vi "Generate Function Call Argument Info.vi"(8 "error in (no error)":errorcluster, 11 "Data Type":variant) -> (0 "error out":errorcluster, 3 "Array":T1[](array[typedef]))   [LabVIEW 2020, in "G-Embedded-Python-Interpreter-Toolkit.lvlib"]
uses:
  G-Embedded-Python-Interpreter-Toolkit.lvlib
  Type Information.ctl
  <vilib>/Utility/Data Type/Type Definitions/Data Type.ctl
  Python Object Reference.ctl
  Python Object Type.ctl
  5ba79b4d-2978-48e4-80f3-d9d30d92ebfd.vi
  <vilib>/Comparison/Equal/Equal Functor/Equal Functor.lvclass
  <vilib>/Utility/Data Type/NI_Data Type.lvlib
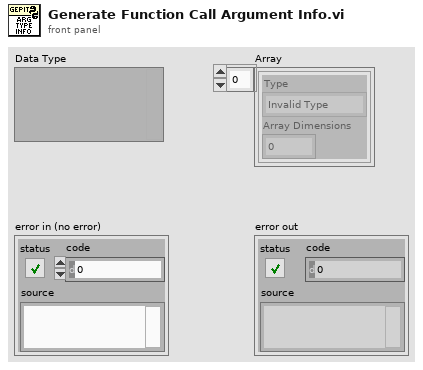
[diagram p1: front panel]
types:
  T1 = typedef "G-Embedded-Python-Interpreter-Toolkit.lvlib/Type Information.ctl" = cluster{"Type":T2, "Array Dimensions":u8}
  T2 = typedef "NI_Data Type.lvlib/Data Type.ctl" = enum8{"Invalid Type", "Void", "I8", "I16", "I32", "I64", "U8", "U16", "U32", "U64", "Single Float", "Double Float", "Extended Float", "Single Complex", "Double Complex", "Extended Complex", "Enum U8", "Enum U16", "Enum U32", "Enum U64", "Single Float With Unit", "Double Float With Unit", "Extended Float With Unit", "Single Complex with Unit", "Double Complex with Unit", "Extended Complex with Unit", "Boolean", "String", "Path", "Picture", "Tag", "Array", "Cluster", "Variant", "LV Variant", "Waveform", "Timestamp", "Digital Waveform", "Digital Data", "ExpressData", "Refnum", "External Data", "VI", "Poly VI", "LabVIEW Class Instance", "Fixed Point", "Set Collection", "Map Collection"}
  T3 = typedef "G-Embedded-Python-Interpreter-Toolkit.lvlib/Python Object Reference.ctl" = refnum<k1>
  T4 = typedef "NI_Data Type.lvlib/Type Definition Info.ctl" = cluster{"Name":string, "Timestamp":u32}
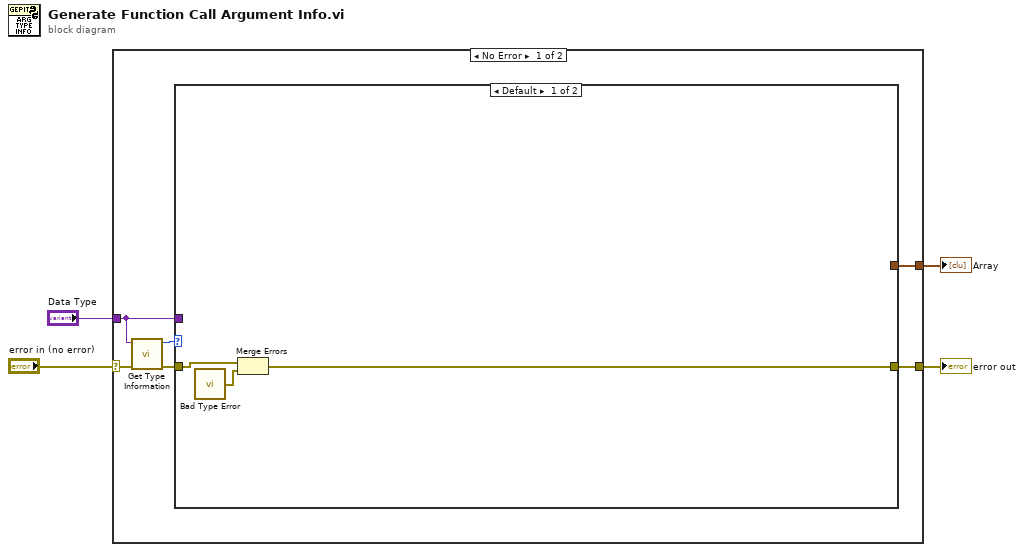
[diagram p0: block diagram]
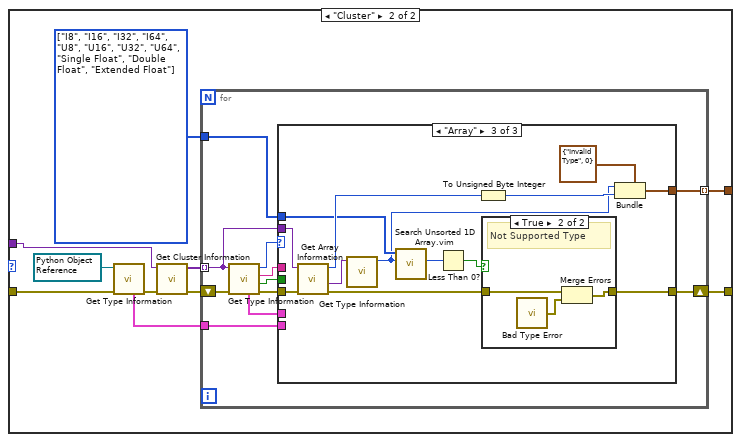
[diagram p2: hidden frame]
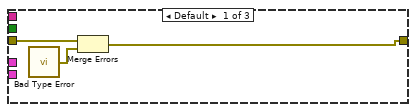
[diagram p3: hidden frame]
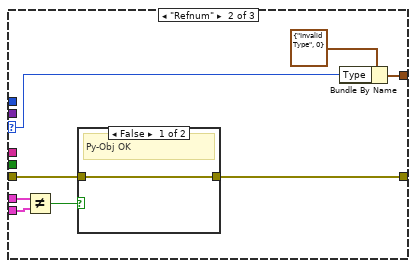
[diagram p4: hidden frame]
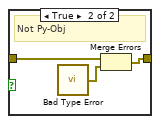
[diagram p5: hidden frame]
diagram:
  n1 = case shown="No Error" "error in (no error)" {
    selector: "error in (no error)" -> [w8 w67]
    tunnel: [w10 w67] -> w4
    tunnel: [w9 _] -> w3
    tunnel: "Data Type" -> [w5 _]
    frame No Error {
      n2 = call <vilib>:"Get Type Information.vi"("error in (no error)"=w8, "variant"=w5) -> ("error out"=w7:errorcluster, "type"=w6:T2)  [unwired: 5 in, 3 out]
      n3 = case shown="Default" w6 {
        tunnel: [w11 w23] -> w10
        tunnel: [_ w22] -> w9
        tunnel: w5 -> [_ w15]
        tunnel: w7 -> [w13 w14]
        frame Default {
          n4 = call "Bad Type Error.vi"() -> ("Unsupported Type Error"=w12:errorcluster)
          n5 = Merge Errors(w13, w12) -> (w11:errorcluster)
        }
        frame "Cluster" {
          w16 = T2[] [enum."I8", enum."I16", enum."I32", enum."I64", enum."U8", enum."U16", enum."U32", enum."U64", enum."Single Float", enum."Double Float", enum."Extended Float"] items=["Invalid Type", "Void", "I8", "I16", "I32", "I64", "U8", "U16", "U32", "U64", "Single Float", "Double Float", "Extended Float", "Single Complex", "Double Complex", "Extended Complex", "Enum U8", "Enum U16", "Enum U32", "Enum U64", "Single Float With Unit", "Double Float With Unit", "Extended Float With Unit", "Single Complex with Unit", "Double Complex with Unit", "Extended Complex with Unit", "Boolean", "String", "Path", "Picture", "Tag", "Array", "Cluster", "Variant", "LV Variant", "Waveform", "Timestamp", "Digital Waveform", "Digital Data", "ExpressData", "Refnum", "External Data", "VI", "Poly VI", "LabVIEW Class Instance", "Fixed Point", "Set Collection", "Map Collection"] ("type")
          w19 = T3 refnum items=["PyObj"] ("Python Object Refnum")
          n6 = call <vilib>:"Get Type Information.vi"("error in (no error)"=w14, "variant"=w19) -> ("error out"=w18:errorcluster, "type definition info"=w17:T4)  [unwired: 5 in, 3 out]
          n7 = call <vilib>:"Get Cluster Information.vi"("error in (no error)"=w18, "variant"=w15) -> ("error out"=w21:errorcluster, "cluster elements"=w20:variant[])  [unwired: 8 in]
          n8 = for {
            tunnel: w20 -> [w33] mode=indexing
            tunnel: [w32] -> w22 mode=indexing
            shift-right: [w25] -> w23
            shift-left: w21 -> [w31]
            tunnel: w17 -> [w26]
            tunnel: w16 -> [w24]
            n9 = call <vilib>:"Get Type Information.vi"("error in (no error)"=w31, "variant"=w33) -> ("error out"=w30:errorcluster, "type definition"=w28:bool, "name"=w29:string, "type"=w34:T2, "type definition info"=w27:T4)  [unwired: 5 in]
            n10 = case shown="\"Array\"" w34 {
              selector: w34 -> [_ w41 _]
              tunnel: w33 -> [_ _ w62]
              tunnel: [_ w42 w59] -> w32
              tunnel: w30 -> [w35 w39 w58]
              tunnel: [w37 w38 w51] -> w25
              tunnel: w29 -> [_ _ _]
              tunnel: w28 -> [_ _ _]
              tunnel: w27 -> [_ w45 _]
              tunnel: w26 -> [_ w44 _]
              tunnel: w24 -> [_ _ w55]
              frame Default {
                n11 = call "Bad Type Error.vi"() -> ("Unsupported Type Error"=w36:errorcluster)
                n12 = Merge Errors(w35, w36) -> (w37:errorcluster)
              }
              frame "Refnum" {
                n13 = Not Equal?(x=w45, y=w44) -> (x != y?=w40:bool)
                n14 = case shown="False" w40 {
                  tunnel: w39 -> [w46 w48]
                  tunnel: [w46 w47] -> w38
                  frame False {
                    # "Py-Obj OK"
                  }
                  frame True {
                    # "Not Py-Obj"
                    n15 = call "Bad Type Error.vi"() -> ("Unsupported Type Error"=w49:errorcluster)
                    n16 = Merge Errors(w48, w49) -> (w47:errorcluster)
                  }
                }
                n17 = Bundle By Name(cluster=T1 {"Type"=enum."Invalid Type", "Array Dimensions"=0} ("Type Info"), "Type"=w41) -> (w42:T1)
              }
              frame "Array" {
                n18 = call <vilib>:"Get Array Information.vi"("error in (no error)"=w58, "variant"=w62) -> ("error out"=w50:errorcluster, "array element data type"=w57:variant, "number of dimensions"=w61:i32)  [unwired: 6 in, 1 out]
                n19 = call <vilib>:"Get Type Information.vi"("variant"=w57) -> ("type"=w54:T2)  [unwired: 6 in, 4 out]
                n20 = call "Search Unsorted 1D Array.vim"("element"=w54, "unsorted 1D array"=w55) -> ("index of element"=w53:i32)  [unwired: 9 in]
                n21 = Less Than 0?(x=w53) -> (x < 0?=w52:bool)
                n22 = To Unsigned Byte Integer(number=w61) -> (unsigned 8bit integer=w60:u8)
                n23 = case shown="True" w52 {
                  tunnel: [w63 w64] -> w51
                  tunnel: w50 -> [w63 w66]
                  frame False {
                    # "Type OK"
                  }
                  frame True {
                    # "Not Supported Type"
                    n24 = call "Bad Type Error.vi"() -> ("Unsupported Type Error"=w65:errorcluster)
                    n25 = Merge Errors(w66, w65) -> (w64:errorcluster)
                  }
                }
                n26 = Bundle(cluster=T1 {"Type"=enum."Invalid Type", "Array Dimensions"=0} ("Type Info"), "Type"=w54, "Array Dimensions"=w60) -> (w59:T1)
              }
            }
          }
        }
      }
    }
    frame Error {
    }
  }
  "error out" <- w4
  "Array" <- w3
